vi "ER2007 Utilities Menu Panel.vi"() -> ()   [LabVIEW 2013]
uses:
  Controls/Global ER2007.vi
panel:
  in  "Test Panel":bool
  in  "Maint":bool
  in  "Setup":bool
  in  "Cal":bool
  out "Copyrightl":string="Program ER2005, Version 1.00, DCI Inc, Copyright 2005, All Rights Reserved"
  # "Utilities Menu"
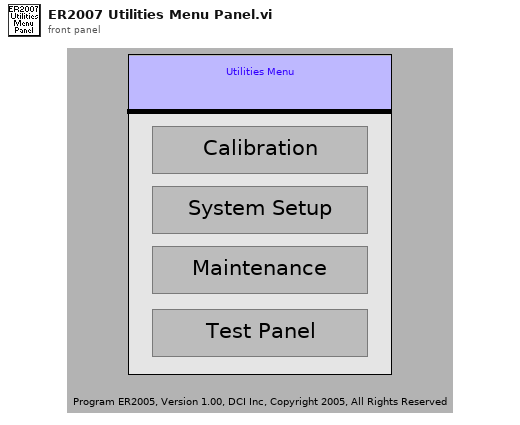
[diagram p1: front panel]
types:
  T1 = cluster{"CurCell":i32, "Cell Data":cluster{"Cell ID":i32, "Cell Status":enum16{"Inactive", "Setup", "Active", "Done"}, "Project":string, "Sample #":string, "Rock Type":string, "Fluid Pair":string, "Rw":dbl, "Rw Temp":dbl, "Length":dbl, "Diameter":dbl, "Porosity":dbl, "Permeability":dbl, "4P":bool, "ElectSpace":dbl, "Frequency":dbl, "Amplitude":dbl, "DAQ Period":u32, "DAQ Units":u16, "Start Time":dbl, "Next Time":dbl, "Datafile":path, "Last Pore Vol":dbl, "Last Pore Xdcr":enum16{"<none>", "Lo Range", "Hi Range"}, "Last Resistor":enum16{"<none>", "Resistor 1", "Resistor 2", "Resistor 3", "Resistor 4", "Resistor 5", "Resistor 6"}, "CurData":dbl[][], "Comment":string}[]}
  T2 = cluster{"Cell ID":i32, "Cell Status":enum16{"Inactive", "Setup", "Active", "Done"}, "Project":string, "Sample #":string, "Rock Type":string, "Fluid Pair":string, "Rw":dbl, "Rw Temp":dbl, "Length":dbl, "Diameter":dbl, "Porosity":dbl, "Permeability":dbl, "4P":bool, "ElectSpace":dbl, "Frequency":dbl, "Amplitude":dbl, "DAQ Period":u32, "DAQ Units":u16, "Start Time":dbl, "Next Time":dbl, "Datafile":path, "Last Pore Vol":dbl, "Last Pore Xdcr":enum16{"<none>", "Lo Range", "Hi Range"}, "Last Resistor":enum16{"<none>", "Resistor 1", "Resistor 2", "Resistor 3", "Resistor 4", "Resistor 5", "Resistor 6"}, "CurData":dbl[][], "Comment":string}[]
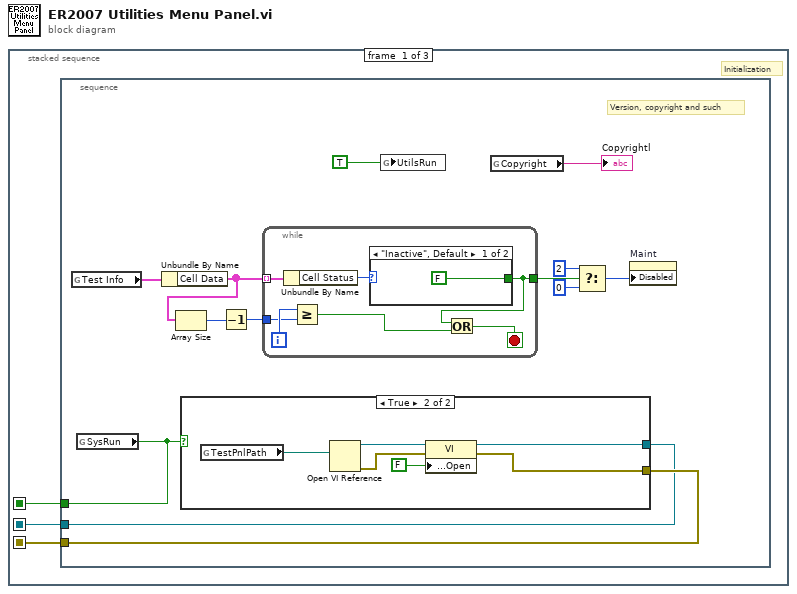
[diagram p0: block diagram]
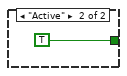
[diagram p2: hidden frame]
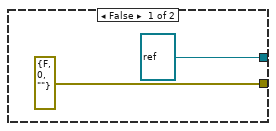
[diagram p3: hidden frame]
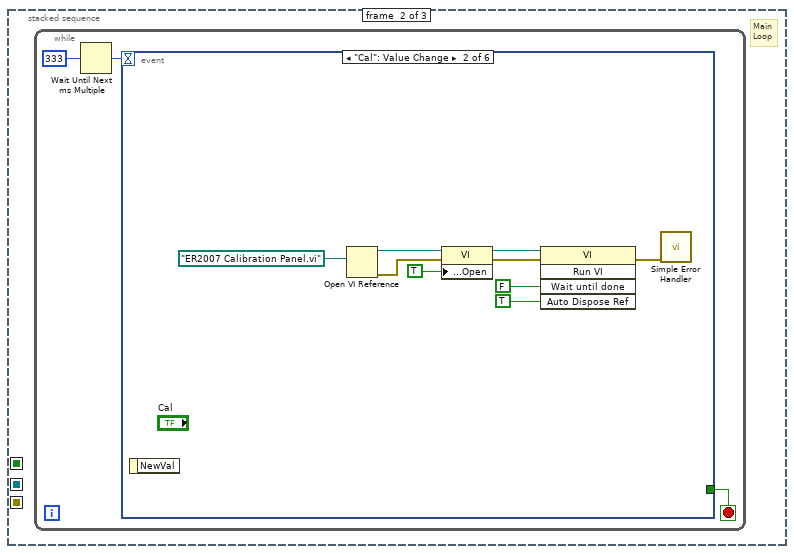
[diagram p4: hidden frame]
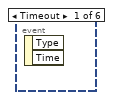
[diagram p5: hidden frame]
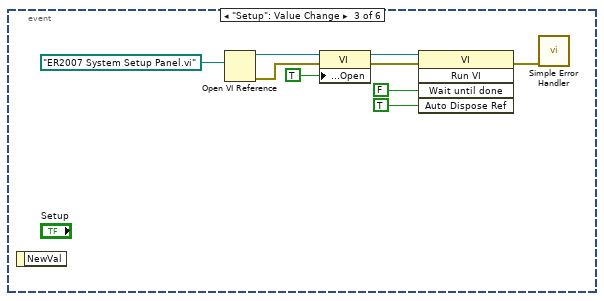
[diagram p6: hidden frame]
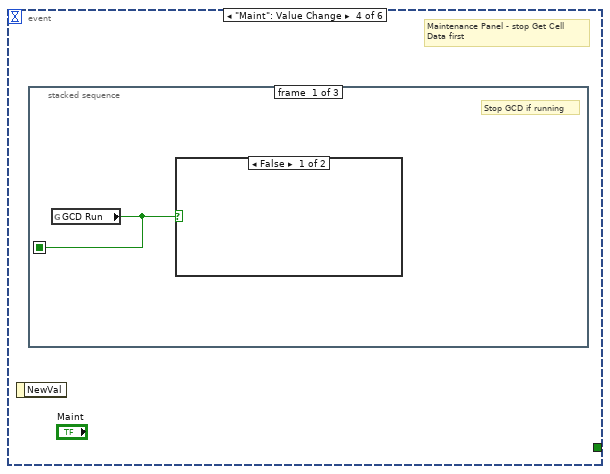
[diagram p7: hidden frame]
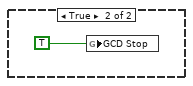
[diagram p8: hidden frame]
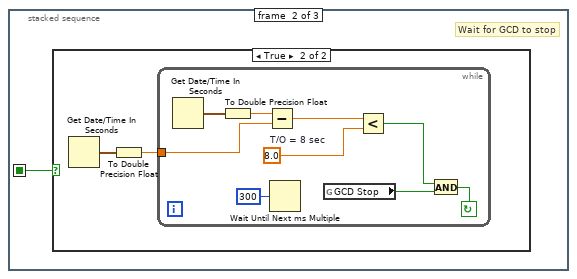
[diagram p9: hidden frame]
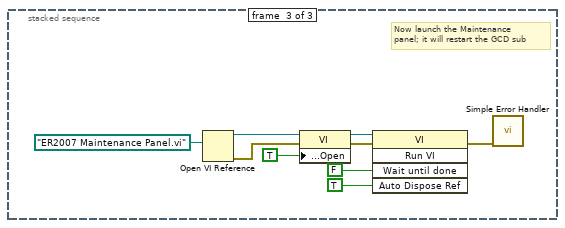
[diagram p11: hidden frame]
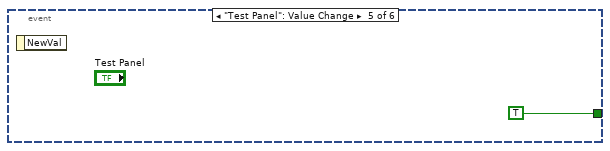
[diagram p12: hidden frame]
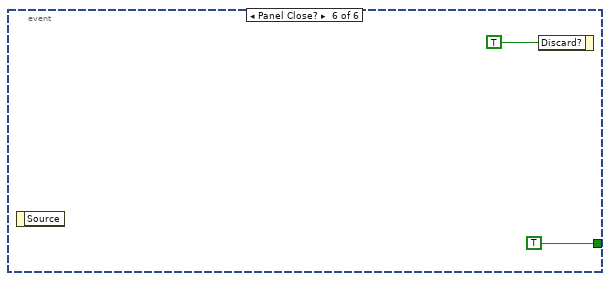
[diagram p13: hidden frame]
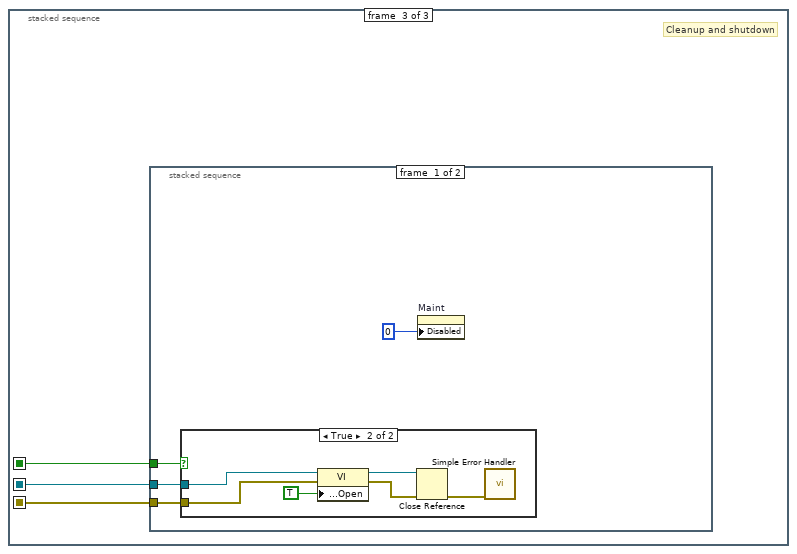
[diagram p14: hidden frame]
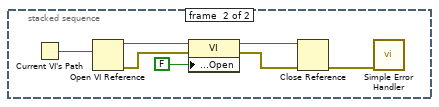
[diagram p16: hidden frame]
diagram:
  n1 = stacked-sequence {
    seq-local: [w3 _ _] -> [_ _ w82]
    seq-local: [w2 _ _] -> [_ _ w81]
    seq-local: [w1 _ _] -> [_ _ w83]
    frame #0 {
      # "Initialization"
      n2 = stacked-sequence {
        tunnel: [w16] -> w3
        tunnel: [w15] -> w2
        tunnel: [w4] -> w1
        frame #0 {
          # "Version, copyright and such"
          n3 = global read "Global ER2007.vi" "Test Info"() -> (w5:T1)
          n4 = global read "Global ER2007.vi" "SysRun"() -> (w4:bool)
          n5 = Unbundle By Name(w5) -> ("Cell Data"=w14:T2)
          n6 = Array Size(array=w14) -> (size(s)=w13:i32)
          n7 = case shown="True" w4 {
            tunnel: [errorcluster {"status"=FALSE, "code"=0, "source"=""} ("error out") w30] -> w16
            tunnel: [refnum<vi> refnum w29] -> w15
            frame False {
            }
            frame True {
              n8 = global read "Global ER2007.vi" "TestPnlPath"() -> (w28:path)
              n9 = Open VI Reference(vi path=w28) -> (vi reference=w33:refnum<vi>, error out=w31:errorcluster)  [unwired: 5 in]
              n10 = property class="VI"(reference=w33, error in=w31, "Front Panel Window:Open"=FALSE) -> (reference out=w29:refnum<vi>, error out=w30:errorcluster)
            }
          }
          n11 = Decrement(x=w13) -> (x-1=w12:i32)
          n12 = while {
            tunnel: w14 -> [w23] mode=indexing
            tunnel: [w19] -> w11
            tunnel: w12 -> [w17]
            i -> [w18]
            stop <- w20 stop-if-true
            n13 = Unbundle By Name(w23) -> ("Cell Status"=w22:enum16{"Inactive", "Setup", "Active", "Done"})
            n14 = Greater Or Equal?(x=w18, y=w17) -> (x >= y?=w21:bool)
            n15 = case shown="\"Inactive\", Default" w22 {
              tunnel: [FALSE TRUE] -> w19
              frame "Inactive", Default {
              }
              frame "Active" {
              }
            }
            n16 = Or(x=w19, y=w21) -> (x .or. y?=w20:bool)
          }
          n17 = global write "Global ER2007.vi" "UtilsRun"(TRUE ("UtilsRun")) -> ()
          n18 = global read "Global ER2007.vi" "Copyright"() -> (→"Copyrightl":string)
          n19 = Select(t=u8 2 ("Disabled"), s=w11, f=u8 0 ("Disabled")) -> (s? t:f=w8:u8)
          n20 = property on="Maint" class="Bool"("Disabled"=w8) -> ()  [unwired: 2 in, 2 out]
        }
      }
    }
    frame #1 {
      # "Main\nLoop"
      n21 = while {
        stop <- w34 stop-if-true
        n22 = Wait Until Next ms Multiple(millisecond multiple=u32 333) -> (millisecond timer value=w35:u32)
        n23 = event shown="[1] \"Cal\": Value Change" {
          selector: _ -> [_ _ _ _ _ _]
          dyn-events: _ -> [_ _ _ _ _ _]
          timeout: w35 -> [_ _ _ _ _ _]
          tunnel: [_ _ _ _ TRUE ("Exit") TRUE ("Exit")] -> w34
          event Timeout {
            n24 = event-data() -> ()  [unwired: 1 in, 2 out]
          }
          event "Cal": Value Change {
            n25 = event-data() -> ()  [unwired: 1 in, 1 out]
            n26 = Open VI Reference(vi path=path "ER2007 Calibration Panel.vi") -> (vi reference=w44:refnum<vi>, error out=w43:errorcluster)  [unwired: 5 in]
            n27 = property class="VI"(reference=w44, error in=w43, "Front Panel Window:Open"=TRUE) -> (reference out=w41:refnum<vi>, error out=w40:errorcluster)
            n28 = invoke class="VI" method="Run VI"(reference=w41, error in=w40, "Wait until done"=FALSE, "Auto Dispose Ref"=TRUE) -> (error out=w37:errorcluster)  [unwired: 1 in, 4 out]
            n29 = call <vilib>:"Simple Error Handler.vi"("error in (no error)"=w37) -> ()  [unwired: 4 in, 5 out]
          }
          event "Setup": Value Change {
            n30 = event-data() -> ()  [unwired: 1 in, 1 out]
            n31 = Open VI Reference(vi path=path "ER2007 System Setup Panel.vi") -> (vi reference=w53:refnum<vi>, error out=w52:errorcluster)  [unwired: 5 in]
            n32 = property class="VI"(reference=w53, error in=w52, "Front Panel Window:Open"=TRUE) -> (reference out=w50:refnum<vi>, error out=w49:errorcluster)
            n33 = invoke class="VI" method="Run VI"(reference=w50, error in=w49, "Wait until done"=FALSE, "Auto Dispose Ref"=TRUE) -> (error out=w46:errorcluster)  [unwired: 1 in, 4 out]
            n34 = call <vilib>:"Simple Error Handler.vi"("error in (no error)"=w46) -> ()  [unwired: 4 in, 5 out]
          }
          event "Maint": Value Change {
            # "Maintenance Panel - stop Get Cell\nData first"
            n35 = event-data() -> ()  [unwired: 1 in, 1 out]
            n36 = stacked-sequence {
              seq-local: [w55 _ _] -> [_ w57 _]
              frame #0 {
                # "Stop GCD if running"
                n37 = global read "Global ER2007.vi" "GCD Run"() -> (w55:bool)
                n38 = case shown="False" w55 {
                  frame False {
                  }
                  frame True {
                    n39 = global write "Global ER2007.vi" "GCD Stop"(TRUE ("GCD Stop")) -> ()
                  }
                }
              }
              frame #1 {
                # "Wait for GCD to stop"
                n40 = case shown="True" w57 {
                  frame False {
                  }
                  frame True {
                    n41 = Get Date/Time In Seconds() -> (seconds since 1Jan1904=w59:timestamp)
                    n42 = To Double Precision Float(number=w59) -> (double precision float=w58:dbl)
                    n43 = while {
                      tunnel: w58 -> [w65]
                      stop <- w63 continue-if-true
                      w64 = 8.0  # T/O = 8 sec
                      n44 = Get Date/Time In Seconds() -> (seconds since 1Jan1904=w67:timestamp)
                      n45 = To Double Precision Float(number=w67) -> (double precision float=w66:dbl)
                      n46 = Subtract(x=w66, y=w65) -> (x-y=w61:dbl)
                      n47 = Wait Until Next ms Multiple(millisecond multiple=u32 300) -> ()  [unwired: 1 out]
                      n48 = global read "Global ER2007.vi" "GCD Stop"() -> (w60:bool)
                      n49 = Less?(x=w61, y=w64) -> (x < y?=w62:bool)
                      n50 = And(x=w62, y=w60) -> (x .and. y?=w63:bool)
                    }
                  }
                }
              }
              frame #2 {
                # "Now launch the Maintenance\npanel; it will restart the GCD sub"
                n51 = Open VI Reference(vi path=path "ER2007 Maintenance Panel.vi") -> (vi reference=w76:refnum<vi>, error out=w75:errorcluster)  [unwired: 5 in]
                n52 = property class="VI"(reference=w76, error in=w75, "Front Panel Window:Open"=TRUE) -> (reference out=w73:refnum<vi>, error out=w72:errorcluster)
                n53 = invoke class="VI" method="Run VI"(reference=w73, error in=w72, "Wait until done"=FALSE, "Auto Dispose Ref"=TRUE) -> (error out=w69:errorcluster)  [unwired: 1 in, 4 out]
                n54 = call <vilib>:"Simple Error Handler.vi"("error in (no error)"=w69) -> ()  [unwired: 4 in, 5 out]
              }
            }
          }
          event "Test Panel": Value Change {
            n55 = event-data() -> ()  [unwired: 1 in, 1 out]
          }
          event Panel Close? {
            n56 = event-data() -> ()  [unwired: 1 in, 1 out]
            n57 = event-data("Discard?"=TRUE) -> ()  [unwired: 1 in, 1 out]
          }
        }
      }
    }
    frame #2 {
      # "Cleanup and shutdown"
      n58 = stacked-sequence {
        tunnel: w83 -> [w87 _]
        tunnel: w82 -> [w86 _]
        tunnel: w81 -> [w85 _]
        frame #0 {
          n59 = case shown="True" w87 {
            tunnel: w86 -> [_ w93]
            tunnel: w85 -> [_ w92]
            frame False {
            }
            frame True {
              n60 = property class="VI"(reference=w92, error in=w93, "Front Panel Window:Open"=TRUE) -> (reference out=w90:refnum<vi>, error out=w89:errorcluster)
              n61 = Close Reference(reference=w90, error in (no error)=w89) -> (error out=w88:errorcluster)
              n62 = call <vilib>:"Simple Error Handler.vi"("error in (no error)"=w88) -> ()  [unwired: 4 in, 5 out]
            }
          }
          n63 = property on="Maint" class="Bool"("Disabled"=u8 0) -> ()  [unwired: 2 in, 2 out]
        }
        frame #1 {
          n64 = Current VI's Path() -> (path=w100:path)
          n65 = Open VI Reference(vi path=w100) -> (vi reference=w99:refnum<vi>, error out=w98:errorcluster)  [unwired: 5 in]
          n66 = property class="VI"(reference=w99, error in=w98, "Front Panel Window:Open"=FALSE) -> (reference out=w96:refnum<vi>, error out=w95:errorcluster)
          n67 = Close Reference(reference=w96, error in (no error)=w95) -> (error out=w94:errorcluster)
          n68 = call <vilib>:"Simple Error Handler.vi"("error in (no error)"=w94) -> ()  [unwired: 4 in, 5 out]
        }
      }
    }
  }
